vi "DataRateTracepoint.vi"(7 "Qbus":refnum<class "Qbus.lvclass">, 10 "data rate u32":u32) -> ()   [LabVIEW 2017]
uses:
  <vilib>/addons/TraceLogger/TraceLogger.lvlib
  <vilib>/addons/Qbus/Qbus.lvclass
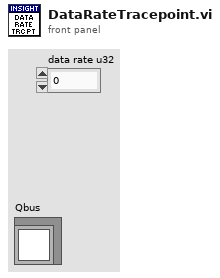
[diagram p1: front panel]
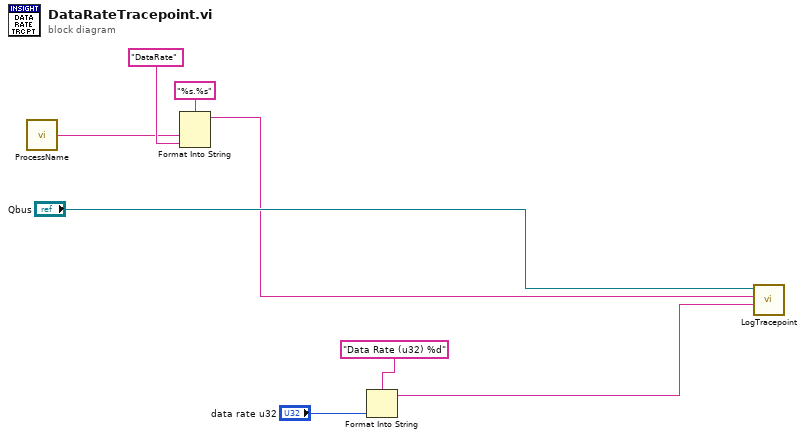
[diagram p0: block diagram]
diagram:
  n1 = call <vilib>:"ProcessName.vi"() -> ("process name"=w1:string)  [unwired: 5 in]
  n2 = Format Into String(format string="%s.%s", w1, "DataRate" ("tracepoint")) -> (resulting string=w4:string)  [unwired: 2 in, 1 out]
  n3 = Format Into String(format string="Data Rate (u32) %d", "data rate u32") -> (resulting string=w2:string)  [unwired: 2 in, 1 out]
  n4 = call <vilib>:"LogTracepoint.vi"("log string"=w2, "tracepoint"=w4, "qbus in"="Qbus") -> ()  [unwired: 7 in, 2 out]
